vi "Substract(I8).vi"(1 "Enable(T)":bool=TRUE, 2 "In":i8, 4 "n":i8=1) -> (6 "Out":i8=1)   [LabVIEW 2013]
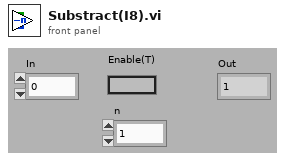
[diagram p1: front panel]
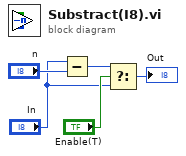
[diagram p0: block diagram]
diagram:
  n1 = Subtract(x="In", y="n") -> (x-y=w1:i8)
  n2 = Select(t=w1, s="Enable(T)", f="In") -> (s? t:f=→"Out":i8)
